vi "Array of strings to multi lined string.vi"(11 "Array in":string[](array[string])) -> (3 "Program":string)   [LabVIEW 2013]
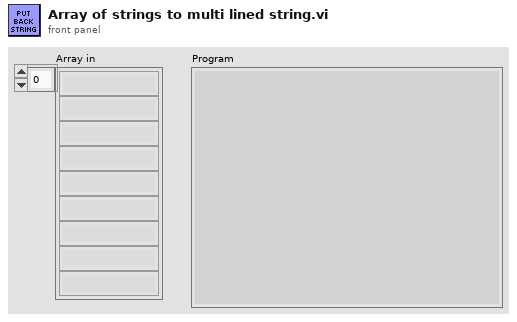
[diagram p1: front panel]
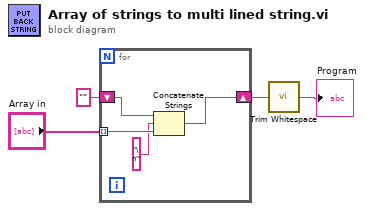
[diagram p0: block diagram]
diagram:
  n1 = for {
    tunnel: "Array in" -> [w7] mode=indexing
    shift-right: [w8] -> w2
    shift-left: "" -> [w6]
    n2 = Concatenate Strings(w6, "\n" ("string"), w7) -> (w8:string)
  }
  n3 = call <vilib>:"Trim Whitespace.vi"("string"=w2) -> ("trimmed string"=→"Program":string)  [unwired: 1 in]
